vi "dump_photon_stream.vi"(5 "acq_mode":T1=2 items=["T2"=2, "T3"=3], 7 "sync":u64[](array[numeric]), 8 "error in (no error)":errorcluster, 9 "channels":u8[](array[numeric]), 10 "photon_records":u64[](array[numeric]), 11 "tt20_logger in":refnum<class "tt20_logger.lvclass">) -> (0 "error out":errorcluster, 3 "tt20_logger out":refnum<class "tt20_logger.lvclass">)   [LabVIEW 2015, in "tt20_logger.lvclass"]
uses:
  tt20_logger.lvclass
  lvoop_dll-master/picoquant_Tmodes.ctl
  tt20_logger.lvclass/tt20_logger.ctl
  <vilib>/UPVI/lvhdf5/dataset.llb/Append Element(s) to Dataset (Variant).vi
  <vilib>/UPVI/lvhdf5/dataset.llb/Append Element(s) to Dataset.xnode
  <vilib>/UPVI/lvhdf5/library.llb/HDF5 Ref.ctl
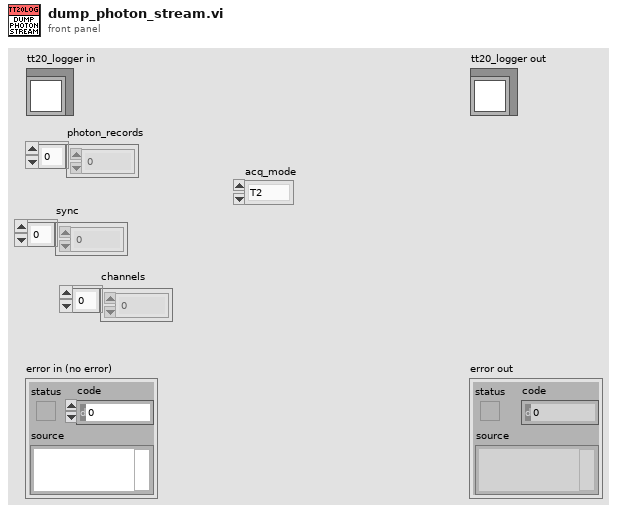
[diagram p1: front panel]
types:
  T1 = typedef "picoquant_Tmodes.ctl" = u16
  T2 = typedef "HDF5 Ref.ctl" = refnum<k1>
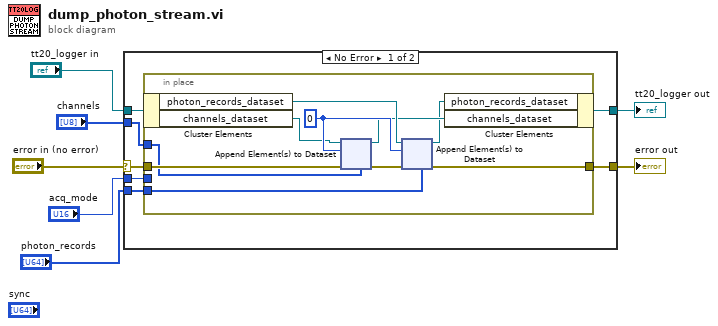
[diagram p0: block diagram]
diagram:
  n1 = case shown="No Error" "error in (no error)" {
    selector: "error in (no error)" -> [w13 w42]
    tunnel: "tt20_logger in" -> [w14 w41]
    tunnel: [w12 w42] -> w3
    tunnel: "acq_mode" -> [w11 _]
    tunnel: [w10 w41] -> w4
    tunnel: "channels" -> [w9 _]
    tunnel: "photon_records" -> [w8 _]
    frame No Error {
      n2 = in-place {
        in-place-border: w13 -> [w23]
        in-place-border: [w21] -> w12
        in-place-border: w11 -> [_]
        in-place-border: w9 -> [w18]
        in-place-border: w8 -> [w17]
        w22 = 0 ("Dimension to Extend (0)")
        n3 = in-place-cluster #1(w14) -> ("photon_records_dataset"=w19:T2, "channels_dataset"=w20:T2)
        n4 = xnode "Append Element(s) to Dataset"("Dimension to Extend (0)"=w22, "HDF5 Dataset Ref"=w20, "error in (no error)"=w23, "Data Element(s)"=w18) -> ("HDF5 Dataset out"=w16:T2, "error out"=w24:errorcluster)  [unwired: 2 out]
        n5 = xnode "Append Element(s) to Dataset"("Dimension to Extend (0)"=w22, "HDF5 Dataset Ref"=w19, "error in (no error)"=w24, "Data Element(s)"=w17) -> ("HDF5 Dataset out"=w15:T2, "error out"=w21:errorcluster)  [unwired: 2 out]
        n6 = in-place-cluster #1("photon_records_dataset"=w15, "channels_dataset"=w16) -> (w10:refnum<class "tt20_logger.lvclass">)
      }
    }
    frame Error {
    }
  }
  "error out" <- w3
  "tt20_logger out" <- w4
